vi "Read Configuration.vi"(8 "error in (no error)":errorcluster) -> (0 "error out":errorcluster, 3 "Ports to Check":T1)   [LabVIEW 2020]
doc: "Reads configuration file and returns ports to check."
uses:
  controls/Ports to Check.ctl
  <vilib>/Utility/config.llb/Read Key (U32).vi
  <vilib>/Utility/config.llb/NI_LVConfig.lvlib
panel:
  out "UDP Values":u32[](array[numeric])
  out "TCP Values":u32[](array[numeric])
  out "Keys":string[][](array[string])
  out "section names":string[](array[string])
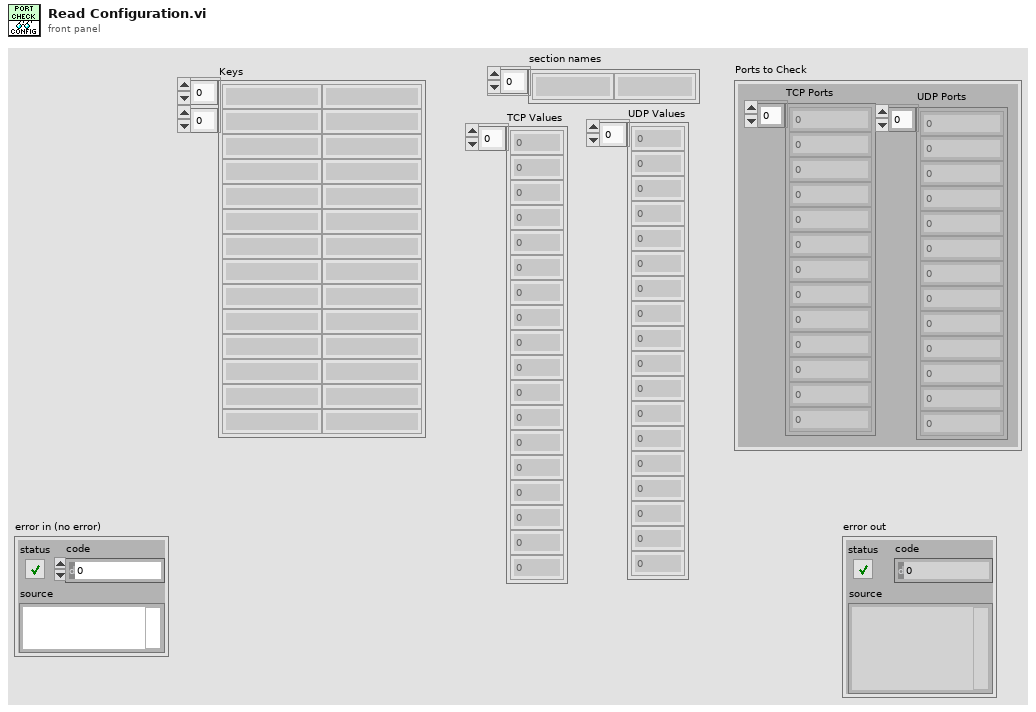
[diagram p1: front panel]
types:
  T1 = typedef "Ports to Check.ctl" = cluster{"TCP Ports":u32[], "UDP Ports":u32[]}
  T2 = typedef "NI_LVConfig.lvlib/Config Data RefNum.ctl" = refnum<k1>
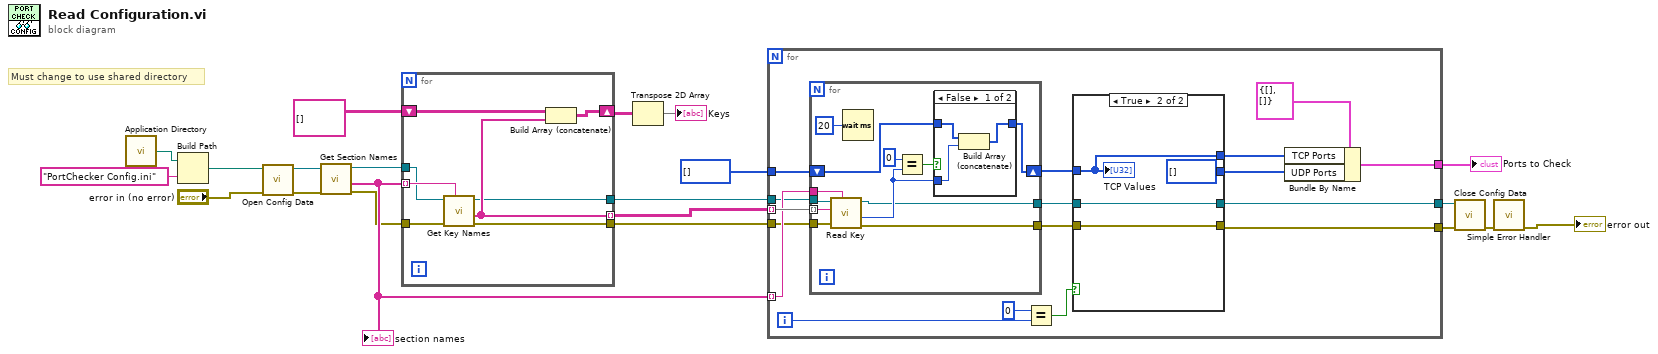
[diagram p0: block diagram]
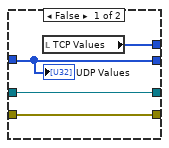
[diagram p2: hidden frame]
diagram:
  # "Must change to use shared directory"
  n1 = call <vilib>:"Application Directory.vi"() -> ("Application Directory"=w21:path)
  n2 = Build Path(base path=w21, name or relative path="PortChecker Config.ini") -> (appended path=w19:path)
  n3 = call <vilib>:"Open Config Data.vi"("error in (no error)"="error in (no error)", "configuration file path"=w19) -> ("error out"=w17:errorcluster, "refnum"=w16:T2)  [unwired: 7 in, 1 out]
  n4 = call <vilib>:"Get Section Names.vi"("error in (no error)"=w17, "refnum"=w16) -> ("error out"=w8:errorcluster, "section names"=w11:string[], "refnum out"=w14:T2)  [unwired: 7 in]
  "section names" <- w11
  n5 = for {
    tunnel: w11 -> [w29] mode=indexing
    tunnel: [w28] -> w10 mode=indexing
    shift-right: [w27] -> w13
    shift-left: string[][] [] -> [w26]
    tunnel: w14 -> [w25]
    tunnel: [w24] -> w9
    tunnel: w8 -> [w23]
    tunnel: [w22] -> w7
    n6 = call <vilib>:"Get Key Names.vi"("section"=w29, "error in (no error)"=w23, "refnum"=w25) -> ("error out"=w22:errorcluster, "key names"=w28:string[], "refnum out"=w24:T2)  [unwired: 5 in, 1 out]
    n7 = Build Array (concatenate)(w26, w28) -> (w27:string[][])
  }
  n8 = Transpose 2D Array(2D array=w13) -> (transposed array=→"Keys":string[][])
  n9 = for {
    tunnel: w11 -> [w45] mode=indexing
    tunnel: w10 -> [w46] mode=indexing
    tunnel: w9 -> [w44]
    tunnel: w7 -> [w43]
    tunnel: u32[] [] -> [w42]
    tunnel: [w34] -> w4
    tunnel: [w32] -> w3
    tunnel: [w30] -> w2
    i -> [w41]
    n10 = for {
      tunnel: w46 -> [w65] mode=indexing
      shift-right: [w58] -> w38
      shift-left: w42 -> [w59]
      tunnel: w45 -> [w64]
      tunnel: w44 -> [w63]
      tunnel: w43 -> [w62]
      tunnel: [w56] -> w33
      tunnel: [w55] -> w31
      n11 = call-poly <vilib>:"Read Key.vi"("section"=w64, "error in (no error)"=w62, "key"=w65, "refnum"=w63) -> ("error out"=w55:errorcluster, "value"=w57:u32, "refnum out"=w56:T2)  [unwired: 4 in, 1 out]
      n12 = Wait (ms)(milliseconds to wait=u32 20) -> ()  [unwired: 1 out]
      n13 = Equal?(x=u32 0, y=w57) -> (x = y?=w61:bool)
      n14 = case shown="False" w61 {
        tunnel: w59 -> [w68 w70]
        tunnel: [w67 w70] -> w58
        tunnel: w57 -> [w69 _]
        frame False {
          n15 = Build Array (concatenate)(w68, w69) -> (w67:u32[])
        }
        frame True {
        }
      }
    }
    n16 = Equal?(x=0 ("y"), y=w41) -> (x = y?=w39:bool)
    n17 = case shown="True" w39 {
      tunnel: w38 -> [w50 w54]
      tunnel: [w50 u32[] []] -> w36
      tunnel: [w47 w54] -> w35
      tunnel: w33 -> [w49 w52]
      tunnel: [w49 w52] -> w32
      tunnel: w31 -> [w48 w51]
      tunnel: [w48 w51] -> w30
      frame False {
        n18 = local read "TCP Values"() -> (w47:u32[])
        "UDP Values" <- w50
      }
      frame True {
        "TCP Values" <- w54
      }
    }
    n19 = Bundle By Name(cluster=T1 {"TCP Ports"=[], "UDP Ports"=[]} ("Ports to Check"), "TCP Ports"=w35, "UDP Ports"=w36) -> (w34:T1)
  }
  "Ports to Check" <- w4
  n20 = call <vilib>:"Close Config Data.vi"("error in (no error)"=w2, "refnum"=w3) -> ("error out"=w6:errorcluster)  [unwired: 8 in, 1 out]
  n21 = call <vilib>:"Simple Error Handler.vi"("error in (no error)"=w6) -> ("error out"=→"error out":errorcluster)  [unwired: 4 in, 4 out]
